vi "Empty Array.vi"() -> (0 "Empty Cluster":variant)   [LabVIEW 2013, in "JKI JSON Serialization.lvlib"]
uses:
  JKI JSON Serialization.lvlib
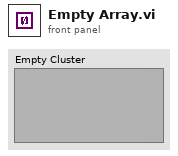
[diagram p1: front panel]
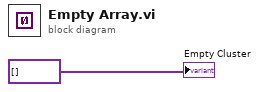
[diagram p0: block diagram]
diagram:
  "Empty Cluster" <- variant[] [] ("Array")
